vi "setMessage.vi"(8 "error in (no error)":errorcluster, 10 "Message.lvclass":refnum<class "Message.lvclass">, 11 "PriorityNode in":refnum<class "PriorityNode.lvclass">) -> (0 "error out":errorcluster, 3 "PriorityNode out":refnum<class "PriorityNode.lvclass">)   [LabVIEW 2009, in "PriorityNode.lvclass"]
uses:
  PriorityNode.lvclass
  Message/Message.lvclass
  PriorityNode.lvclass/PriorityNode.ctl
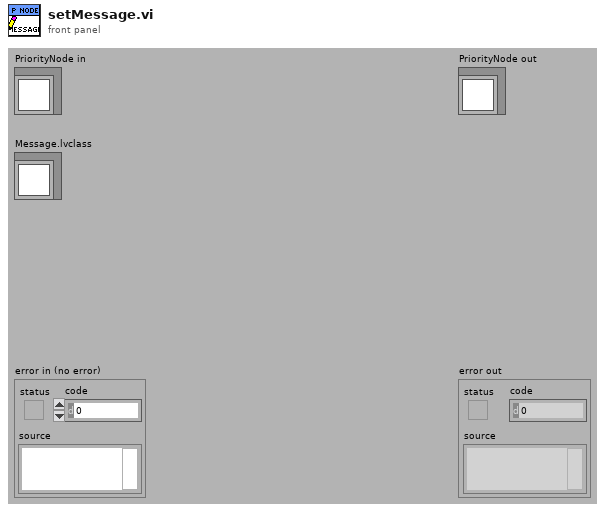
[diagram p1: front panel]
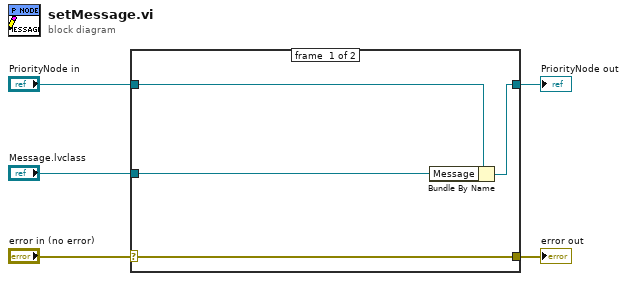
[diagram p0: block diagram]
diagram:
  n1 = case shown="No Error" "error in (no error)" {
    selector: "error in (no error)" -> [w9 w10]
    tunnel: [w9 w10] -> w4
    tunnel: [w7 w11] -> w2
    tunnel: "PriorityNode in" -> [w8 w11]
    tunnel: "Message.lvclass" -> [w6 _]
    frame #0 {
      n2 = Bundle By Name(cluster=w8, "Message"=w6) -> (w7:refnum<class "PriorityNode.lvclass">)
    }
    frame #1 {
    }
  }
  "error out" <- w4
  "PriorityNode out" <- w2
